vi "Overall_M14_Sim.vi"() -> ()   [LabVIEW 2019]
uses:
  Utility_VIs/Joystick_Controls.ctl
  Program Files (x86)/National Instruments/LabVIEW 2019/Targets/NI/RT/vi.lib/Rock Robotics/WPI/DriverStation/WPI_DriverStationRobotMode2.ctl
panel:
  in  "Robot Mode":T1
  in  "Joystick_In":T2
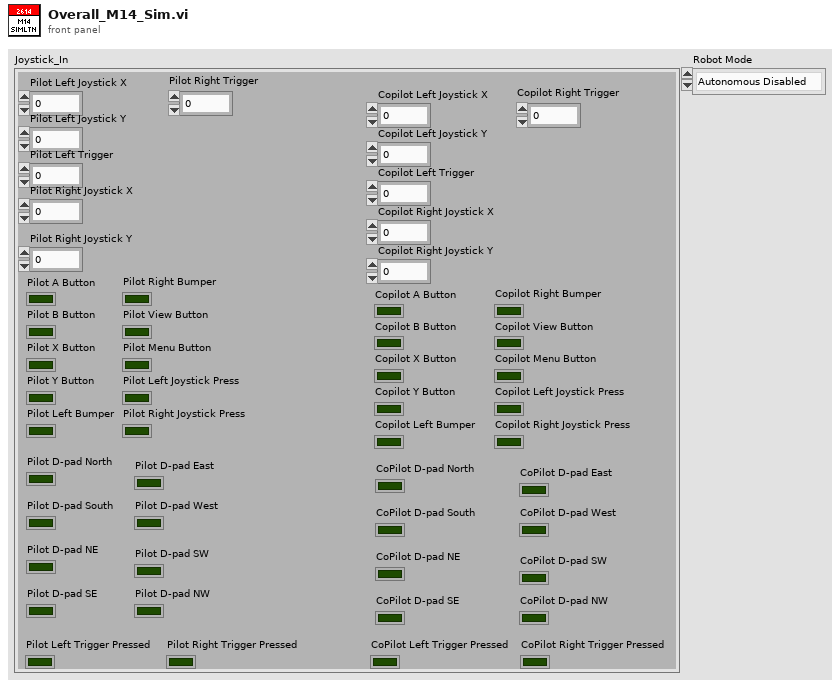
[diagram p1: front panel]
types:
  T1 = typedef "WPI_DriverStationRobotMode2.ctl" = enum16{"Autonomous Disabled", "Autonomous Enabled", "Teleop Disabled", "Teleop Enabled", "Disconnected", "Finish", "Test Disabled", "Test Enabled", "Emergency Stopped"}
  T2 = typedef "Joystick_Controls.ctl" = cluster{"Pilot Left Joystick X":dbl, "Pilot Left Joystick Y":dbl, "Pilot A Button":bool, "Pilot B Button":bool, "Pilot X Button":bool, "Pilot Y Button":bool, "Pilot Left Bumper":bool, "Pilot Right Bumper":bool, "Pilot View Button":bool, "Pilot Menu Button":bool, "Pilot Left Joystick Press":bool, "Pilot Right Joystick Press":bool, "Pilot Left Trigger":dbl, "Pilot Right Joystick X":dbl, "Pilot Right Joystick Y":dbl, "Pilot Right Trigger":dbl, "Copilot Left Joystick X":dbl, "Copilot Left Joystick Y":dbl, "Copilot A Button":bool, "Copilot B Button":bool, "Copilot X Button":bool, "Copilot Y Button":bool, "Copilot Left Bumper":bool, "Copilot Right Bumper":bool, "Copilot View Button":bool, "Copilot Menu Button":bool, "Copilot Left Joystick Press":bool, "Copilot Right Joystick Press":bool, "Copilot Left Trigger":dbl, "Copilot Right Joystick X":dbl, "Copilot Right Joystick Y":dbl, "Copilot Right Trigger":dbl, "Pilot D-pad North":bool, "Pilot D-pad South":bool, "Pilot D-pad East":bool, "Pilot D-pad West":bool, "Pilot D-pad NE ":bool, "Pilot D-pad SE":bool, "Pilot D-pad SW":bool, "Pilot D-pad NW":bool, "CoPilot D-pad North":bool, "CoPilot D-pad South":bool, "CoPilot D-pad East":bool, "CoPilot D-pad West":bool, "CoPilot D-pad NE":bool, "CoPilot D-pad SE":bool, "CoPilot D-pad SW":bool, "CoPilot D-pad NW":bool, "Pilot Left Trigger Pressed":bool, "Pilot Right Trigger Pressed":bool, "CoPilot Left Trigger Pressed":bool, "CoPilot Right Trigger Pressed":bool}
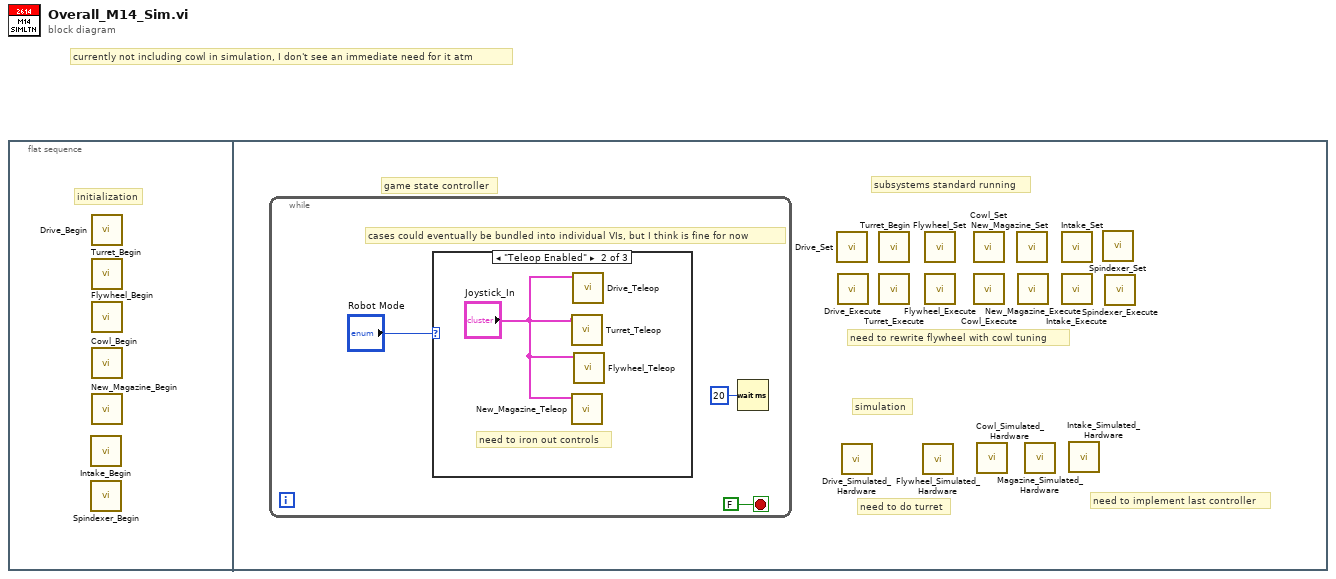
[diagram p0: block diagram]
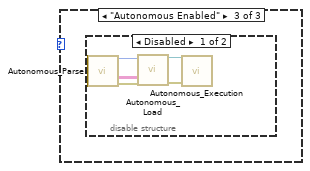
[diagram p3: hidden frame]
diagram:
  # "currently not including cowl in simulation, I don't see an immediate need for it atm"
  n1 = flat-sequence {
    frame #0 {
      # "initialization"
      n2 = call "Intake_Begin.vi"() -> ()  [unwired: 12 in]
      n3 = call "Spindexer_Begin.vi"() -> ()  [unwired: 12 in]
      n4 = call "Drive_Begin.vi"() -> ()  [unwired: 12 in]
      n5 = call "Turret_Begin.vi"() -> ()  [unwired: 12 in]
      n6 = call "Flywheel_Begin.vi"() -> ()  [unwired: 12 in]
      n7 = call "Cowl_Begin.vi"() -> ()  [unwired: 12 in]
      n8 = call "New_Magazine_Begin.vi"() -> ()  [unwired: 12 in]
    }
    frame #1 {
      # "need to implement last controller"
      # "need to do turret"
      # "simulation"
      # "subsystems standard running"
      # "game state controller"
      # "need to rewrite flywheel with cowl tuning"
      n9 = while {
        stop <- FALSE stop-if-true
        # "cases could eventually be bundled into individual VIs, but I think is fine for now"
        n10 = case shown="\"Teleop Enabled\"" "Robot Mode" {
          frame "Autonomous Disabled", Default {
          }
          frame "Teleop Enabled" {
            # "need to iron out controls"
            n11 = call "Turret_Teleop.vi"("Joystick_IN"="Joystick_In") -> ()  [unwired: 11 in]
            n12 = call "New_Magazine_Teleop.vi"("Joystick_In"="Joystick_In") -> ()  [unwired: 11 in]
            n13 = call "Drive_Teleop.vi"("Joystick_In"="Joystick_In") -> ()  [unwired: 11 in]
            n14 = call "Flywheel_Teleop.vi"("Joystick_IN"="Joystick_In") -> ()  [unwired: 11 in]
          }
          frame "Autonomous Enabled" {
            n15 = disable-structure shown="Disabled" {
              frame Disabled {
                n16 = call "Autonomous_Parse.vi"() -> ("Number of Commands"=w5:i32, "Inputs"=w9:string[][], "errror out"=w8:errorcluster)  [unwired: 9 in, 4 out]
                n17 = call "Autonomous_Load.vi"("Number of Commands"=w5, "Inputs"=w9, "error in"=w8) -> ("Queue_Key"=w6:refnum<queue>, "errror out"=w7:errorcluster)  [unwired: 10 in, 1 out]
                n18 = call "Autonomous_Execution.vi"("error in"=w7, "Queue Key"=w6) -> ()  [unwired: 9 in, 1 out]
              }
              frame Enabled {
              }
            }
          }
        }
        n19 = Wait (ms)(milliseconds to wait=u32 20) -> ()  [unwired: 1 out]
      }
      n20 = call "Drive_Set.vi"() -> ()  [unwired: 12 in]
      n21 = call "Drive_Execute.vi"() -> ()  [unwired: 12 in]
      n22 = call "Drive_Simulated_Hardware.vi"() -> ()  [unwired: 12 in]
      n23 = call "Turret_Begin.vi"() -> ()  [unwired: 12 in]
      n24 = call "Turret_Execute.vi"() -> ()  [unwired: 12 in]
      n25 = call "Flywheel_Simulated_Hardware.vi"() -> ()  [unwired: 12 in]
      n26 = call "Flywheel_Set.vi"() -> ()  [unwired: 12 in]
      n27 = call "Flywheel_Execute.vi"() -> ()  [unwired: 12 in]
      n28 = call "Cowl_Set.vi"() -> ()  [unwired: 12 in]
      n29 = call "Cowl_Execute.vi"() -> ()  [unwired: 12 in]
      n30 = call "Cowl_Simulated_Hardware.vi"() -> ()  [unwired: 12 in]
      n31 = call "New_Magazine_Set.vi"() -> ()  [unwired: 12 in]
      n32 = call "New_Magazine_Execute.vi"() -> ()  [unwired: 12 in]
      n33 = call "Magazine_Simulated_Hardware.vi"() -> ()  [unwired: 12 in]
      n34 = call "Intake_Set.vi"() -> ()  [unwired: 12 in]
      n35 = call "Intake_Execute.vi"() -> ()  [unwired: 12 in]
      n36 = call "Intake_Simulated_Hardware.vi"() -> ()  [unwired: 12 in]
      n37 = call "Spindexer_Set.vi"() -> ()  [unwired: 12 in]
      n38 = call "Spindexer_Execute.vi"() -> ()  [unwired: 12 in]
    }
  }
